vi "StatusWarning.vi"(10 "Text.Text":string, 11 "String in":refnum<vi>) -> ()   [LabVIEW 2020]
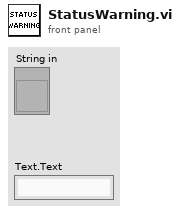
[diagram p1: front panel]
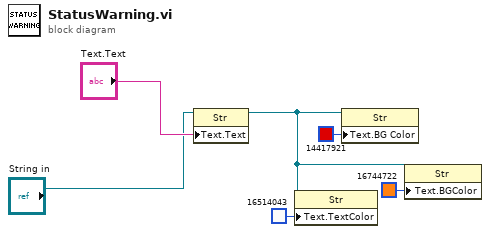
[diagram p0: block diagram]
diagram:
  n1 = property class="Str"(reference="String in", "Text.Text"="Text.Text") -> (reference out=w5:refnum<vi>)  [unwired: 1 in, 1 out]
  n2 = property class="Str"(reference=w5, "Text.TextColor"=u32 16514043 ("Text.Text Colors:Text Color")) -> ()  [unwired: 1 in, 2 out]
  n3 = property class="Str"(reference=w5, "Text.BG Color"=u32 14417921 ("Text.Colors:BG Color")) -> ()  [unwired: 1 in, 2 out]
  n4 = property class="Str"(reference=w5, "Text.BGColor"=u32 16744722 ("Text.Text Colors:BG Color")) -> ()  [unwired: 1 in, 2 out]
